vi "Configure Trigger.vi"(8 "error in":errorcluster, 11 "Scope PXI CFG in":refnum<class "Scope PXI CFG.lvclass">) -> (0 "error out":errorcluster, 3 "Scope PXI CFG out":refnum<class "Scope PXI CFG.lvclass">)   [LabVIEW 2023, in "Scope.lvlib" / "Scope PXI.lvlib" / "Scope PXI CFG.lvclass"]
uses:
  Scope PXI CFG.lvclass
  <instrlib>/niScope/Controls/niScope trigger slope.ctl
  <instrlib>/niScope/Controls/niScope trigger source digital.ctl
  Scope PXI CFG.lvclass/Scope PXI CFG.ctl
  Configuration Base/Configuration Base.lvclass/Configuration Base.ctl
  795efc06-cdc5-4534-8f89-f6f4812d0b8b.vi
  84d48f8e-c3f0-4191-b0b5-590cc168e0e0.vi
  d6385bd9-32f1-4e86-8d66-f1f6b280b9ec.vi
  4b4b6126-2405-414b-91da-33c74864ffaf.vi
  733de5b7-6890-4c28-a56b-02f88581e263.vi
  <vilib>/JDP Science/JSONtext/Next JSON Value.vi
  <vilib>/JDP Science/JSONtext/String Subset.vi
  <vilib>/JDP Science/JSONtext/Parsing/Advance past next JSON Value (inlined COPY).vi
  <vilib>/JDP Science/JSONtext/Parsing/Advance past whitespace.vi
  <vilib>/JDP Science/JSONtext/Parsing/Advance past String.vi
  <vilib>/JDP Science/JSONtext/Parsing/Advance past Number.vi
  <vilib>/JDP Science/JSONtext/Parsing/Advance past Line Ending.vi
  <vilib>/JDP Science/JSONtext/Parsing/Parse Full Path or Item Name.vi
  <vilib>/JDP Science/JSONtext/Parsing/Advance past Array.vi
  <vilib>/JDP Science/JSONtext/Parsing/Advance past Object.vi
  <vilib>/JDP Science/JSONtext/support/Error Cluster From Code.vi
  <vilib>/JDP Science/JSONtext/Offset/Find Item Locations by Path.vi
  <vilib>/JDP Science/JSONtext/JSON text to Variant.vi
  <vilib>/Utility/error.llb/Error Cluster From Error Code.vi
  <instrlib>/niScope/Configure/Trigger/niScope Configure Trigger Digital.vi
  <instrlib>/niScope/Configure/Trigger/niScope Configure Trigger Immediate.vi
  <instrlib>/niScope/Configure/Trigger/niScope Configure Trigger Software.vi
  <vilib>/JDP Science/JSONtext/LVClass Serializer/JSONtext LVClass Serializer.lvclass
  <vilib>/ErrorRing/Error Ring.xnode
  Configuration Base/Configuration Base.lvclass
  <vilib>/JDP Science/JSONtext/JSONtext.lvlib
panel:
  out "trigger source":T1="VAL_RTSI_0" caption="trigger source (RTSI 0)"
  out "trigger slope":T2 items=["Positive", "Negative"]
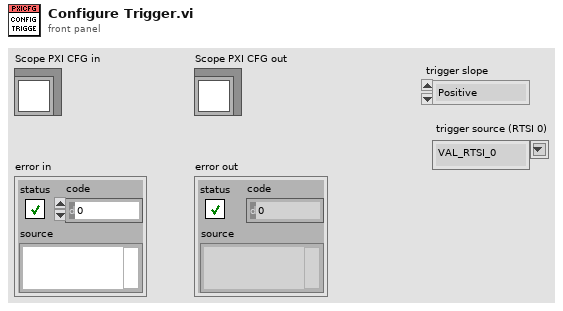
[diagram p1: front panel]
types:
  T1 = typedef "niScope trigger source digital.ctl" = string
  T2 = typedef "niScope trigger slope.ctl" = i32
  T3 = typedef "LVStringsAndValuesArrayTypeDef_I32.ctl" = cluster{"String":string, "Value":i32}[]
  T4 = typedef "LVComboBoxStrsAndValuesArrayTypeDef.ctl" = cluster{"String":string, "Value":string}[]
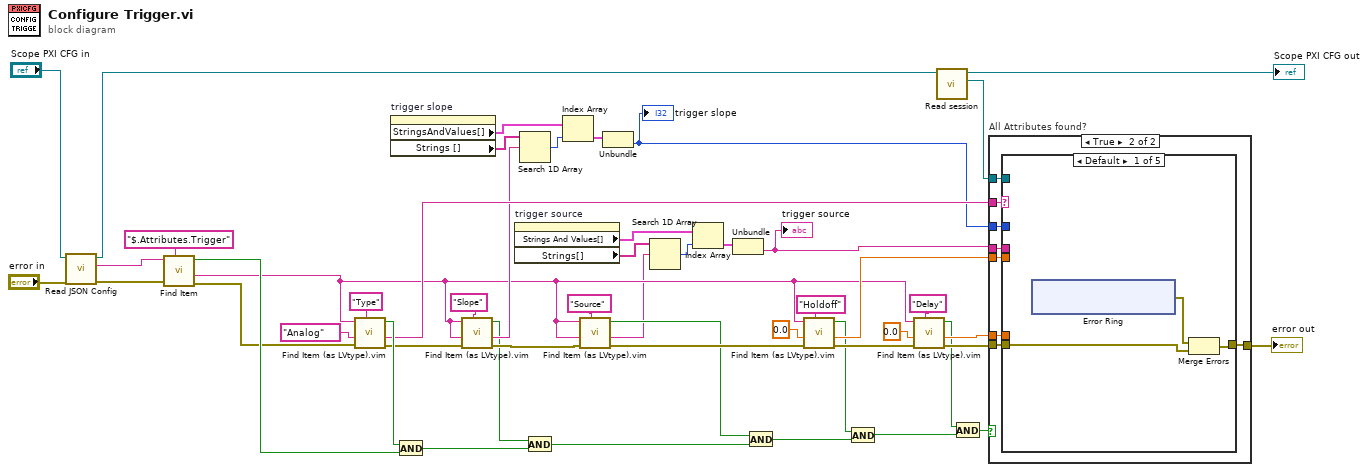
[diagram p0: block diagram]
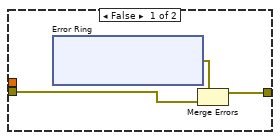
[diagram p2: hidden frame]
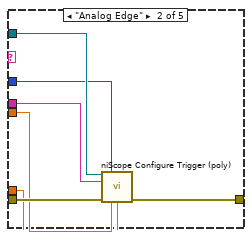
[diagram p3: hidden frame]
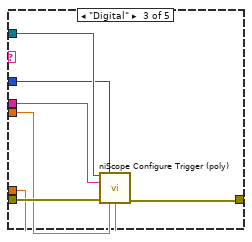
[diagram p4: hidden frame]
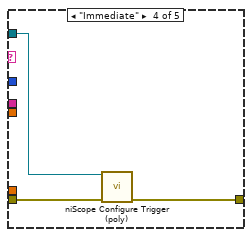
[diagram p5: hidden frame]
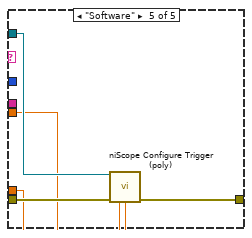
[diagram p6: hidden frame]
diagram:
  n1 = call "Read JSON Config.vi"("error in"="error in", "object in"="Scope PXI CFG in") -> ("error out"=w49:errorcluster, "<JSON>Config"=w46:string, "object out"=w47:refnum<class "Scope PXI CFG.lvclass">)  [unwired: 7 in]
  n2 = call <vilib>:"Find Item.vi"("$Path or Item Name"="$.Attributes.Trigger", "error in (no error)"=w49, "JSON"=w46) -> ("error out"=w44:errorcluster, "<JSON>"=w7:string, "Found"=w45:bool)  [unwired: 5 in, 1 out]
  n3 = call "Find Item (as LVtype).vim"("$Path or Item Name"="Type", "error in (no error)"=w44, "Data Type and Default Value"="Analog" ("Type"), "JSON"=w7) -> ("error out"=w21:errorcluster, "Data"=w28:string, "Found"=w37:bool)  [unwired: 4 in, 1 out]
  n4 = property on="trigger slope" class="Ring (strict)"() -> ("StringsAndValues[]"=w10:T3, "Strings []"=w18:string[])  [unwired: 2 in, 2 out]
  n5 = And(x=w37, y=w45) -> (x .and. y?=w15:bool)
  n6 = call "Find Item (as LVtype).vim"("$Path or Item Name"="Slope", "error in (no error)"=w21, "Data Type and Default Value"=w7, "JSON"=w7) -> ("error out"=w20:errorcluster, "Data"=w17:string, "Found"=w16:bool)  [unwired: 4 in, 1 out]
  n7 = property on="trigger source" class="CmbBox (strict)"() -> ("Strings And Values[]"=w4:T4, "Strings[]"=w6:string[])  [unwired: 2 in, 2 out]
  n8 = Search 1D Array(1D array=w18, element=w17) -> (index of element=w11:i32)  [unwired: 1 in]
  n9 = And(x=w16, y=w15) -> (x .and. y?=w22:bool)
  n10 = Index Array(array=w10, index=w11) -> (element=w9:cluster{"String":string, "Value":i32})
  n11 = call "Find Item (as LVtype).vim"("$Path or Item Name"="Source", "error in (no error)"=w20, "Data Type and Default Value"=w7, "JSON"=w7) -> ("error out"=w40:errorcluster, "Data"=w2:string, "Found"=w36:bool)  [unwired: 4 in, 1 out]
  n12 = Unbundle(w9) -> ("Value"=w8:i32)  [unwired: 1 out]
  "trigger slope" <- w8
  n13 = Search 1D Array(1D array=w6, element=w2) -> (index of element=w5:i32)  [unwired: 1 in]
  n14 = Index Array(array=w4, index=w5) -> (element=w3:cluster{"String":string, "Value":string})
  n15 = Unbundle(w3) -> ("Value"=w1:string)  [unwired: 1 out]
  "trigger source" <- w1
  n16 = And(x=w36, y=w22) -> (x .and. y?=w34:bool)
  n17 = call "Find Item (as LVtype).vim"("$Path or Item Name"="Holdoff", "error in (no error)"=w40, "Data Type and Default Value"=0.0, "JSON"=w7) -> ("error out"=w39:errorcluster, "Data"=w38:dbl, "Found"=w35:bool)  [unwired: 4 in, 1 out]
  n18 = And(x=w35, y=w34) -> (x .and. y?=w12:bool)
  n19 = call "Find Item (as LVtype).vim"("$Path or Item Name"="Delay", "error in (no error)"=w39, "Data Type and Default Value"=0.0, "JSON"=w7) -> ("error out"=w26:errorcluster, "Data"=w25:dbl, "Found"=w13:bool)  [unwired: 4 in, 1 out]
  n20 = call "Read session.vi"("Scope PXI CFG in"=w47) -> ("session"=w48:refnum<k15>, "Scope PXI CFG out"=→"Scope PXI CFG out":refnum<class "Scope PXI CFG.lvclass">)  [unwired: 8 in, 1 out]
  n21 = And(x=w13, y=w12) -> (x .and. y?=w14:bool)
  n22 = case "All Attributes found?" shown="True" w14 {
    tunnel: w26 -> [w51 w65]
    tunnel: w1 -> [_ w63]
    tunnel: [w52 w64] -> w31
    tunnel: w38 -> [_ w62]
    tunnel: w48 -> [_ w66]
    tunnel: w28 -> [_ w61]
    tunnel: w25 -> [_ w60]
    tunnel: w8 -> [_ w59]
    frame False {
      n23 = xnode "Error Ring"() -> ("error out"=w53:errorcluster)
      n24 = Merge Errors(w53, w51) -> (w52:errorcluster)
    }
    frame True {
      n25 = case shown="Default" w61 {
        tunnel: w66 -> [_ w79 w85 w89 w96]
        tunnel: w65 -> [w67 w81 w88 w91 w95]
        tunnel: [w69 w80 w87 w90 w94] -> w64
        tunnel: w63 -> [_ w78 w86 _ _]
        tunnel: w62 -> [_ w76 w84 _ w93]
        tunnel: w60 -> [_ w77 w83 _ w92]
        tunnel: w59 -> [_ w75 w82 _ _]
        frame Default {
          n26 = xnode "Error Ring"() -> ("error out"=w68:errorcluster)
          n27 = Merge Errors(w68, w67) -> (w69:errorcluster)
        }
        frame "Analog Edge" {
          n28 = call-poly <instrlib>:"niScope Configure Trigger (poly).vi"("instrument handle"=w79, "trigger slope"=w75, "trigger source"=w78, "error in"=w81, "trigger holdoff"=w76, "trigger delay"=w77) -> ("error out"=w80:errorcluster)  [unwired: 8 in, 1 out]
        }
        frame "Digital" {
          n29 = call-poly <instrlib>:"niScope Configure Trigger (poly).vi"("instrument handle"=w85, "trigger slope"=w82, "trigger source"=w86, "error in"=w88, "trigger holdoff"=w84, "trigger delay"=w83) -> ("error out"=w87:errorcluster)  [unwired: 8 in, 1 out]
        }
        frame "Immediate" {
          n30 = call-poly <instrlib>:"niScope Configure Trigger (poly).vi"("instrument handle"=w89, "error in"=w91) -> ("error out"=w90:errorcluster)  [unwired: 12 in, 1 out]
        }
        frame "Software" {
          n31 = call-poly <instrlib>:"niScope Configure Trigger (poly).vi"("instrument handle"=w96, "error in"=w95, "trigger holdoff"=w93, "trigger delay"=w92) -> ("error out"=w94:errorcluster)  [unwired: 10 in, 1 out]
        }
      }
    }
  }
  "error out" <- w31
